vi "Main.vi"(7 "Is Simulated?":bool, 8 "error in":errorcluster, 9 ">>ErrorQ":refnum<queue>, 10 ">>ControllerQ":refnum<queue>, 11 ">>EventHandlers":refnum<user-event>) -> (0 "error out":errorcluster)   [LabVIEW 2020, in "Controller.lvlib"]
doc: "This is a template for creating new VIs for the owning library"
uses:
  Controller.lvlib
  Error Handler/Controls/Error QMsg.ctl
  Support/Controls/Project Modules.ctl
  Controls/Controller QMsg.ctl
  Support/Controls/Project Event Msg.ctl
  Support/Controls/Project Events.ctl
  Controls/Operational Loop Data.ctl
  Support/Support.lvlib
  Controls/Module Event Msg.ctl
  Error Handler/ErrorHandler.lvlib
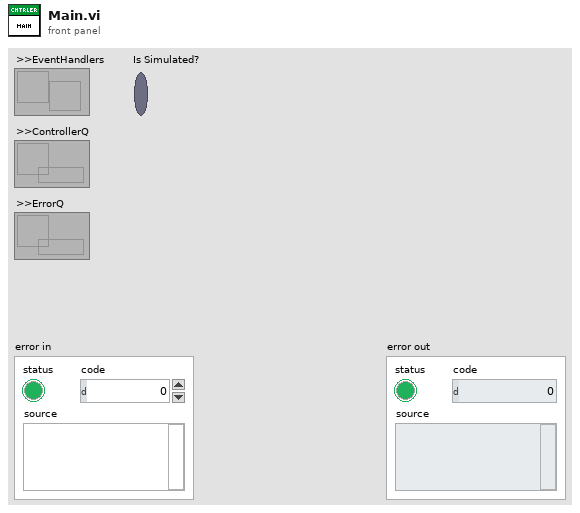
[diagram p1: front panel]
types:
  T1 = typedef "Controller.lvlib/Controller QMsg.ctl" = cluster{"Command":string, "Data":variant}
  T2 = typedef "Controller.lvlib/Operational Loop Data.ctl" = cluster{"Is Simulated?":bool, "Current State":string}
  T3 = typedef "Controller.lvlib/Module Messaging Structures.ctl" = cluster{">>EventHandlers":refnum<user-event>, ">>ErrorQ":refnum<queue>, ">>ControllerQ":refnum<queue>}
  T4 = typedef "Controller.lvlib/Module Event Msg.ctl" = cluster{"Command":string, "Data":variant}
  T5 = typedef "Support.lvlib/Project Events.ctl" = enum16{"Stop", "Initialize", "Elevator Call"}
  T6 = typedef "Support.lvlib/Project Event Msg.ctl" = cluster{"Command":string, "Data":variant, "Events":T5}
  T7 = cluster{"Direction is Up?":bool, "Current Floor":i32}
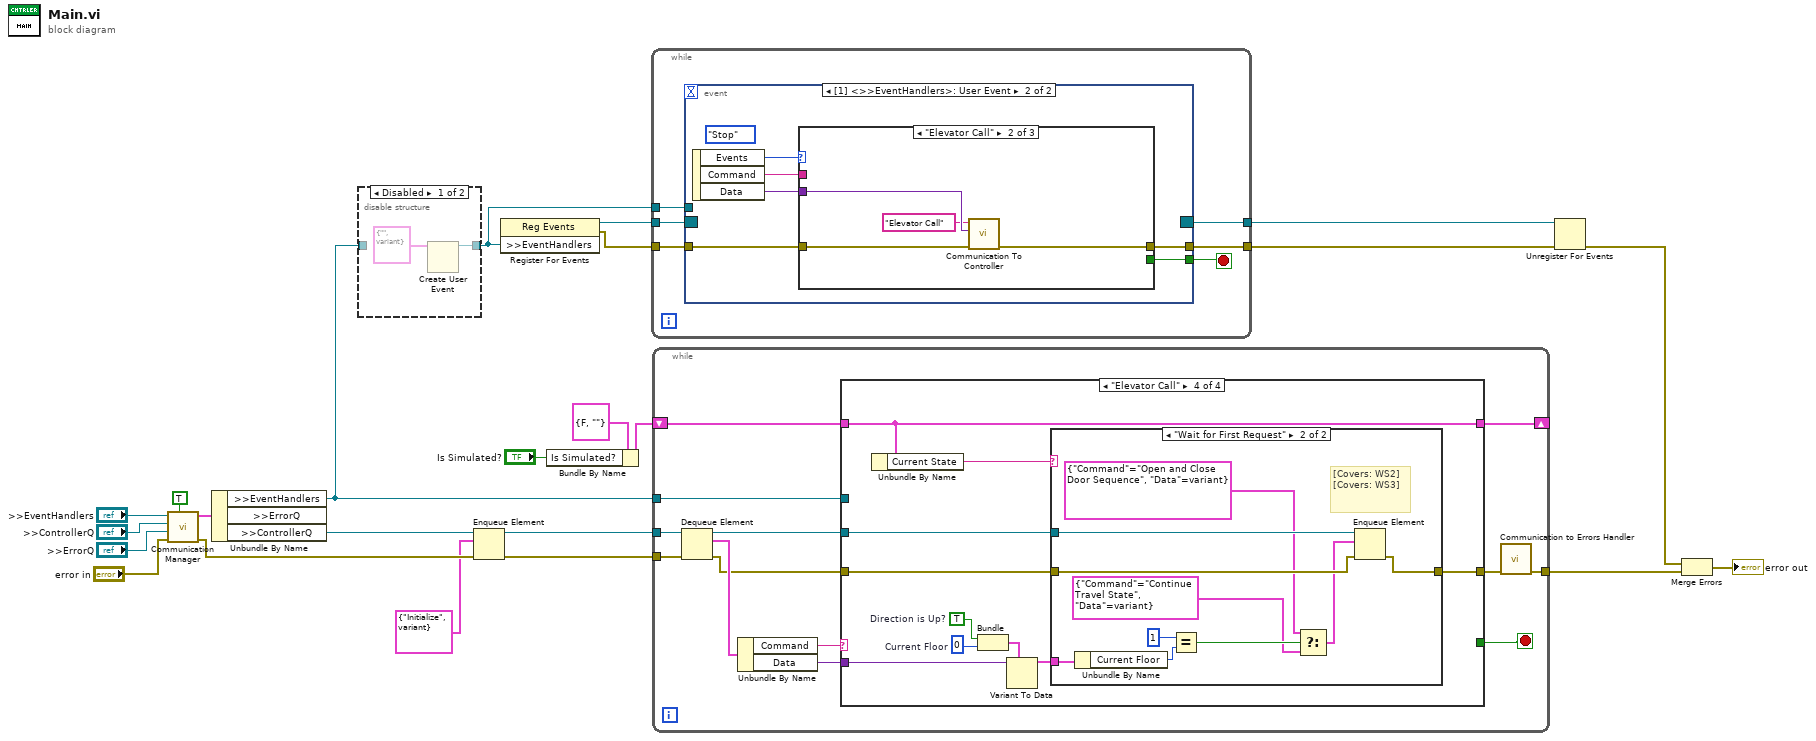
[diagram p0: block diagram]
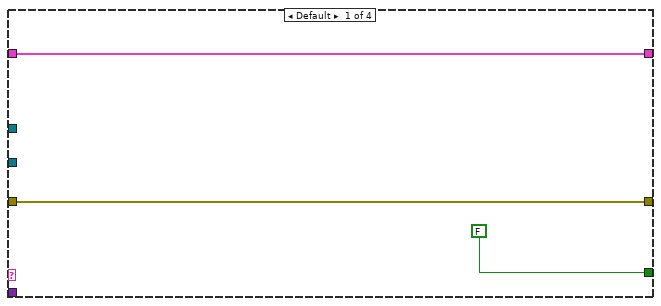
[diagram p3: hidden frame]
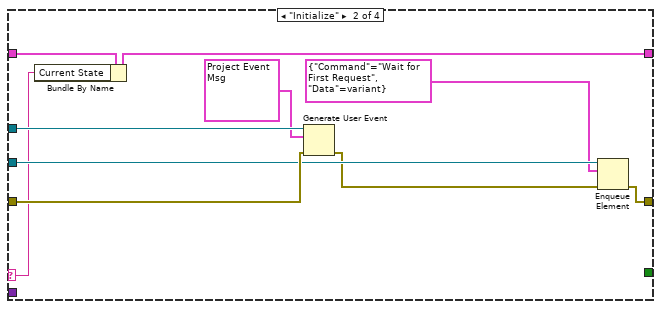
[diagram p4: hidden frame]
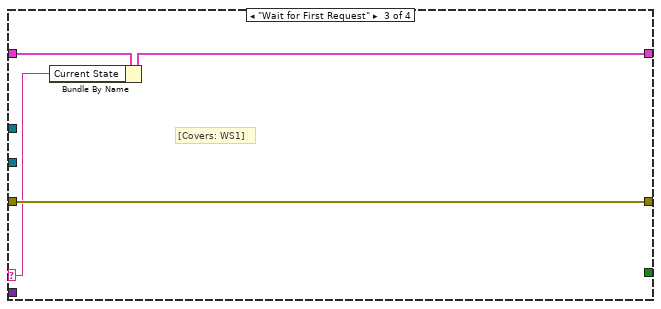
[diagram p5: hidden frame]
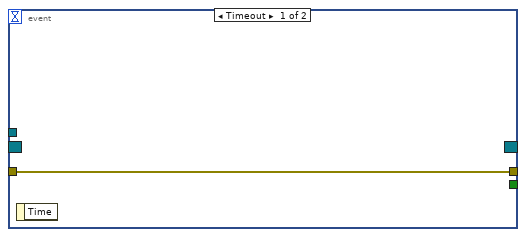
[diagram p7: hidden frame]
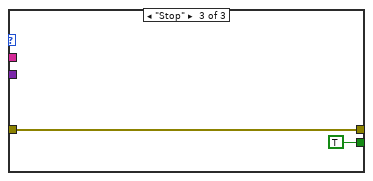
[diagram p9: hidden frame]
diagram:
  n1 = call "Communication Manager.vi"("Load?"=TRUE, "error in"="error in", ">>ErrorQ"=">>ErrorQ", ">>ControllerQ"=">>ControllerQ", ">>EventHandlers"=">>EventHandlers") -> ("error out"=w3:errorcluster, "Messaging Structures"=w18:T3)  [unwired: 5 in]
  n2 = Unbundle By Name(w18) -> (">>EventHandlers"=w7:refnum<user-event>, ">>ControllerQ"=w5:refnum<queue>)  [unwired: 1 out]
  n3 = disable-structure shown="Disabled" {
    disable-tunnel: w7 -> [_ w26]
    disable-tunnel: [w24 w26] -> w6
    frame Disabled {
      n4 = Create User Event(user event datatype=T4 {"Command"="", "Data"=variant} ("QMessage")) -> (user event=w24:refnum<user-event>)  [unwired: 1 in, 1 out]
    }
    frame Enabled {
    }
  }
  n5 = Enqueue Element(queue=w5, element=T1 {"Command"="Initialize", "Data"=variant}, error in (no error)=w3) -> (queue out=w4:refnum<queue>, error out=w2:errorcluster)  [unwired: 1 in, 1 out]
  n6 = register-events(w6) -> (reference out=w17:refnum<event-registration>, error out=w15:errorcluster)  [unwired: 2 in]
  n7 = Bundle By Name(cluster=T2 {"Is Simulated?"=FALSE, "Current State"=""} ("Operation Loop Data"), "Is Simulated?"="Is Simulated?") -> (w9:T2)
  n8 = while {
    tunnel: w6 -> [w32]
    tunnel: w17 -> [w31]
    tunnel: [w30] -> w16
    tunnel: w15 -> [w29]
    tunnel: [w28] -> w14
    stop <- w27 stop-if-true
    n9 = event shown="[1] <>>EventHandlers>: User Event" {
      selector: w31 -> [_ _]
      dyn-events: [_ _] -> w30
      timeout: _ -> [_ _]
      tunnel: w32 -> [_ _]
      tunnel: w29 -> [w33 w39]
      tunnel: [w33 w38] -> w28
      tunnel: [_ w36] -> w27
      event Timeout {
        n10 = event-data() -> ()  [unwired: 1 in, 1 out]
      }
      event User Event {
        (unwired) Project_Events."Stop" ("Events")
        n11 = event-data() -> ("Events"=w37:T5, "Command"=w35:string, "Data"=w34:variant)  [unwired: 1 in]
        n12 = case shown="\"Elevator Call\"" w37 {
          tunnel: w39 -> [w40 w44 w46]
          tunnel: [w40 w43 w46] -> w38
          tunnel: [_ _ TRUE] -> w36
          tunnel: w35 -> [_ _ _]
          tunnel: w34 -> [_ w42 _]
          frame Default {
          }
          frame "Elevator Call" {
            n13 = call "Communication To Controller.vi"("error in"=w44, "Data"=w42, "Command"="Elevator Call") -> ("error out"=w43:errorcluster)  [unwired: 8 in]
          }
          frame "Stop" {
          }
        }
      }
    }
  }
  n14 = while {
    tunnel: w4 -> [w59]
    tunnel: w7 -> [w52]
    tunnel: w2 -> [w58]
    tunnel: [w50] -> w12
    shift-right: [w48] -> _
    shift-left: w9 -> [w49]
    stop <- w54 stop-if-true
    n15 = Dequeue Element(queue=w59, error in (no error)=w58) -> (queue out=w47:refnum<queue>, element=w57:T1, error out=w53:errorcluster)  [unwired: 1 in, 1 out]
    n16 = Unbundle By Name(w57) -> ("Command"=w56:string, "Data"=w55:variant)
    n17 = case shown="\"Elevator Call\"" w56 {
      selector: w56 -> [_ w64 w75 _]
      tunnel: w55 -> [_ _ _ w86]
      tunnel: [FALSE _ _ _] -> w54
      tunnel: w53 -> [w62 w71 w76 w79]
      tunnel: [w62 w67 w76 w80] -> w51
      tunnel: w52 -> [_ w72 _ _]
      tunnel: w49 -> [w61 w65 w74 w82]
      tunnel: [w61 w63 w73 w82] -> w48
      tunnel: w47 -> [_ w69 _ w77]
      frame Default {
      }
      frame "Initialize" {
        n18 = Bundle By Name(cluster=w65, "Current State"=w64) -> (w63:T2)
        n19 = Generate User Event(user event=w72, event data cluster=T6 {"Command"="", "Data"=variant, "Events"=enum."Initialize"} ("event data"), error in=w71) -> (error out=w68:errorcluster)  [unwired: 1 in, 1 out]
        n20 = Enqueue Element(queue=w69, element=T1 {"Command"="Wait for First Request", "Data"=variant}, error in (no error)=w68) -> (error out=w67:errorcluster)  [unwired: 1 in, 2 out]
      }
      frame "Wait for First Request" {
        # "[Covers: WS1]"
        n21 = Bundle By Name(cluster=w74, "Current State"=w75) -> (w73:T2)
      }
      frame "Elevator Call" {
        w84 = 0  # Current Floor
        w85 = TRUE  # Direction is Up?
        n22 = Unbundle By Name(w82) -> ("Current State"=w81:string)
        n23 = Bundle("Direction is Up?"=w85, "Current Floor"=w84) -> (w83:T7)  [unwired: 1 in]
        n24 = Variant To Data(type=w83, Variant=w86) -> (data=w78:T7)  [unwired: 1 in, 1 out]
        n25 = case shown="\"Wait for First Request\"" w81 {
          tunnel: [w87 w95] -> w80
          tunnel: w79 -> [w87 w96]
          tunnel: w78 -> [_ w94]
          tunnel: w77 -> [_ w97]
          frame Default {
            # "Elevator Call event was fired up, \nbut we are not in the wait for request state"
          }
          frame "Wait for First Request" {
            # "[Covers: WS2] \n[Covers: WS3]"
            n26 = Unbundle By Name(w94) -> ("Current Floor"=w93:i32)
            n27 = Equal?(x=1, y=w93) -> (x = y?=w91:bool)
            n28 = Select(t=T1 {"Command"="Open and Close Door Sequence", "Data"=variant} ("element"), s=w91, f=T1 {"Command"="Continue Travel State", "Data"=variant} ("element")) -> (s? t:f=w90:T1)
            n29 = Enqueue Element(queue=w97, element=w90, error in (no error)=w96) -> (error out=w95:errorcluster)  [unwired: 1 in, 2 out]
          }
        }
      }
    }
    n30 = call "Communication to Errors Handler.vi"("error in"=w51) -> ("error out"=w50:errorcluster)  [unwired: 10 in]
  }
  n31 = Unregister For Events(event registration refnum=w16, error in=w14) -> (error out=w13:errorcluster)
  n32 = Merge Errors(w13, w12) -> (→"error out":errorcluster)
